vi "CMN_PathParams2Path.vi"(9 "const vars":string[](array[string])=["_CONFPATH_", "_LOGPATH_", "_MODPATH_", "_COMMPATH_", "_MACROPATH_"], 10 "Path In":path, 11 "Dabatase name":string="DBS") -> (2 "Path out":path)   [LabVIEW 2016]
uses:
  DBSHAND/private/vis/DatabaseHand_Element_Get(string).vi
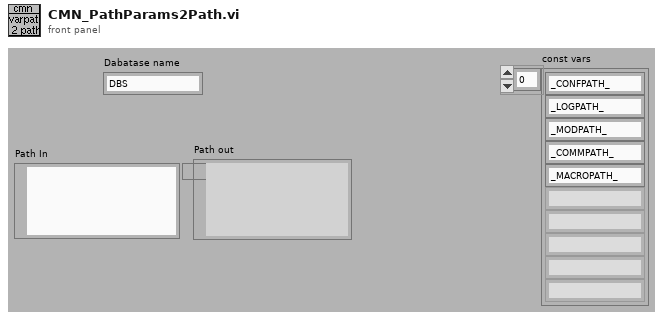
[diagram p1: front panel]
types:
  T1 = typedef "DatabaseHand_RefNum.ctl" = refnum<vi>
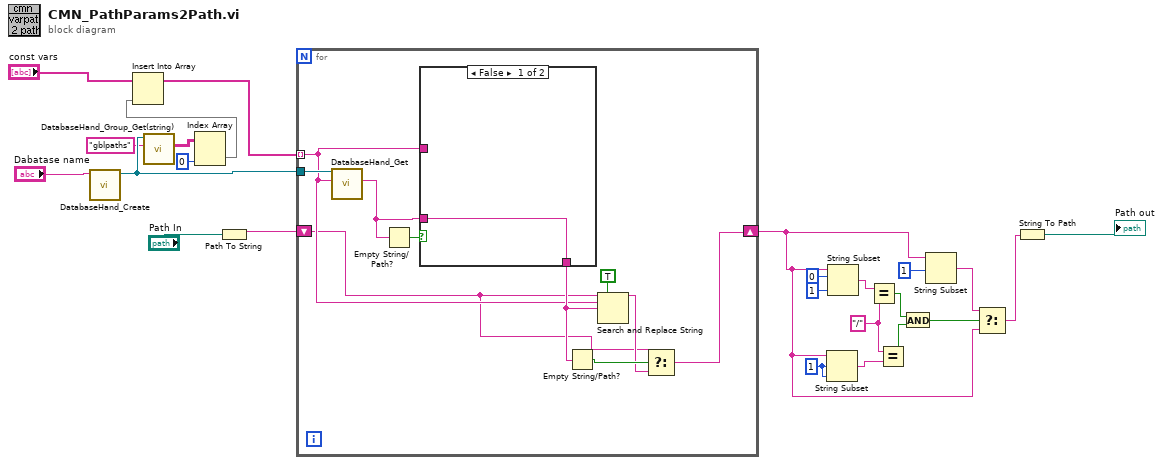
[diagram p0: block diagram]
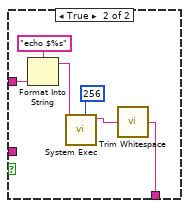
[diagram p2: hidden frame]
diagram:
  w10 = 1 ("offset (0)")
  w8 = "/" ("y")
  n1 = call "DatabaseHand_Create.vi"("Name"="Dabatase name") -> ("Database RefNum out"=w19:T1)  [unwired: 1 in, 9 out]
  n2 = call "DatabaseHand_Group_Get(string).vi"("group"="gblpaths", "Database RefNum in"=w19) -> ("group array"=w17:string[][])  [unwired: 1 in, 8 out]
  n3 = Index Array(array=w17, index (col)=0 ("disabled index (col)")) -> (element=w16:string[])  [unwired: 1 in]
  n4 = Insert Into Array(array="const vars", new element=w16) -> (w15:string[])  [unwired: 1 in]
  n5 = Path To String(path="Path In") -> (string=w22:string)
  n6 = for {
    tunnel: w15 -> [w29] mode=indexing
    tunnel: w19 -> [w34]
    shift-right: [w27] -> w3
    shift-left: w22 -> [w28]
    n7 = call-poly "DatabaseHand_Get.vi"("name"=w29, "Database RefNum in"=w34) -> ("value"=w25:string)  [unwired: 3 in, 6 out]
    n8 = Empty String/Path?(string/path=w25) -> (empty?=w26:bool)
    n9 = case shown="False" w26 {
      tunnel: [w35 w37] -> w32
      tunnel: w29 -> [_ w39]
      tunnel: w25 -> [w35 _]
      frame False {
      }
      frame True {
        n10 = Format Into String(format string="echo $%s", w39) -> (resulting string=w36:string)  [unwired: 2 in, 1 out]
        n11 = call <vilib>:"System Exec.vi"("expected output size  (4096)"=u32 256, "command line"=w36) -> ("standard output"=w40:string)  [unwired: 5 in, 4 out]
        n12 = call <vilib>:"Trim Whitespace.vi"("string"=w40) -> ("trimmed string"=w37:string)  [unwired: 1 in]
      }
    }
    n13 = Empty String/Path?(string/path=w32) -> (empty?=w31:bool)
    n14 = Search and Replace String(replace all?=TRUE ("replace all? (F)"), input string=w28, search string=w29, replace string=w32) -> (result string=w30:string)  [unwired: 1 in, 6 out]
    n15 = Select(t=w28, s=w31, f=w30) -> (s? t:f=w27:string)
  }
  n16 = String Subset(string=w3, offset (0)=w10, length (rest)=w10) -> (substring=w9:string)
  n17 = String Subset(string=w3, offset (0)=0, length (rest)=1 ("length (rest)")) -> (substring=w11:string)
  n18 = Equal?(x=w11, y=w8) -> (x = y?=w7:bool)
  n19 = Equal?(x=w8, y=w9) -> (x = y?=w6:bool)
  n20 = And(x=w7, y=w6) -> (x .and. y?=w4:bool)
  n21 = String Subset(string=w3, offset (0)=1) -> (substring=w1:string)  [unwired: 1 out]
  n22 = Select(t=w1, s=w4, f=w3) -> (s? t:f=w5:string)
  n23 = String To Path(string=w5) -> (path=→"Path out":path)
